vi "AMI_Check_Queue.vi"(7 "error in (no error)":errorcluster, 10 "queue":refnum<queue>) -> (0 "error out":errorcluster, 1 "AMI_Control":T1, 3 "New Entries?":bool)   [LabVIEW 2019]
uses:
  AMI/AMI_Control.ctl
panel:
  out "Numeric":i32
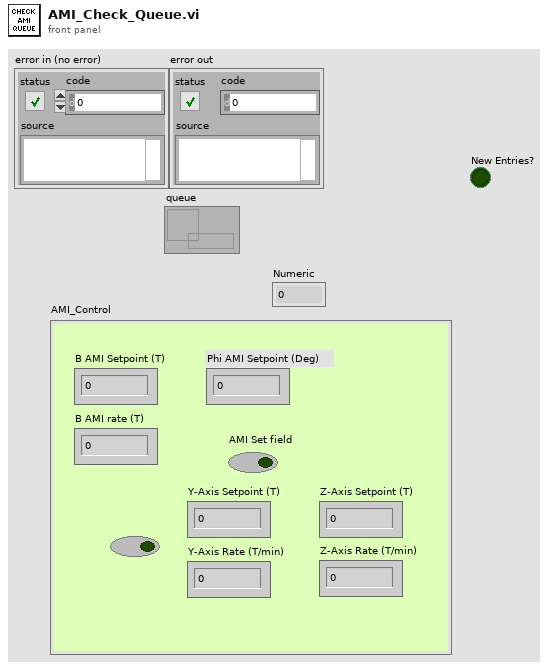
[diagram p1: front panel]
types:
  T1 = typedef "AMI_Control.ctl" = cluster{"B AMI rate (T)":dbl, "AMI Set field":bool, "B AMI Setpoint (T)":dbl, "Phi AMI Setpoint (Deg) ":dbl, "Switch Heater":bool, "Y-Axis Setpoint (T)":dbl, "Y-Axis Rate (T/min)":dbl, "Z-Axis Setpoint (T)":dbl, "Z-Axis Rate (T/min)":dbl}
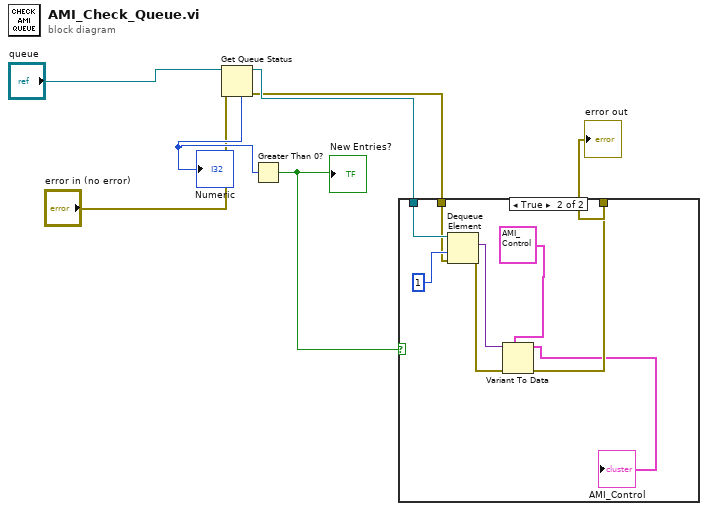
[diagram p0: block diagram]
diagram:
  n1 = Get Queue Status(queue="queue", error in (no error)="error in (no error)") -> (queue out=w6:refnum<queue>, error out=w4:errorcluster, # elements in queue=w7:i32)  [unwired: 1 in, 5 out]
  "Numeric" <- w7
  n2 = Greater Than 0?(x=w7) -> (x > 0?=w5:bool)
  "New Entries?" <- w5
  n3 = case shown="True" w5 {
    tunnel: w6 -> [_ w14]
    tunnel: w4 -> [w8 w13]
    tunnel: [w8 w11] -> w2
    frame False {
    }
    frame True {
      n4 = Dequeue Element(queue=w14, timeout in ms (-1)=1, error in (no error)=w13) -> (element=w15:variant, error out=w12:errorcluster)  [unwired: 2 out]
      n5 = Variant To Data(error in=w12, type=T1 {"B AMI rate (T)"=0.0, "AMI Set field"=FALSE, "B AMI Setpoint (T)"=0.0, "Phi AMI Setpoint (Deg) "=0.0, "Switch Heater"=FALSE, "Y-Axis Setpoint (T)"=0.0, "Y-Axis Rate (T/min)"=0.0, "Z-Axis Setpoint (T)"=0.0, "Z-Axis Rate (T/min)"=0.0} ("AMI_Control 2"), Variant=w15) -> (data=→"AMI_Control":T1, error out=w11:errorcluster)
    }
  }
  "error out" <- w2
